vi "Normalize Time Array.vi"(11 "Array Input":dbl[][](array[numeric])) -> (3 "Array Output":dbl[][](array[numeric]))   [LabVIEW 2020]
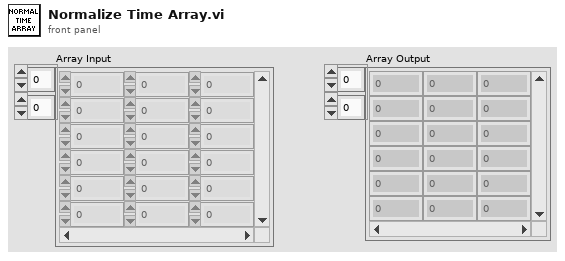
[diagram p1: front panel]
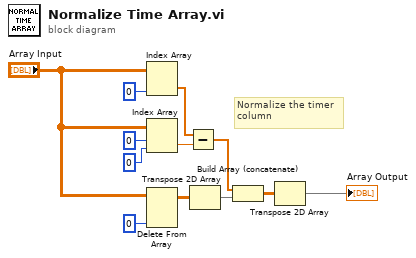
[diagram p0: block diagram]
diagram:
  # "Normalize the timer\ncolumn"
  n1 = Index Array(array="Array Input", index (col)=0 ("disabled index (col)")) -> (element=w7:dbl[])  [unwired: 1 in]
  n2 = Index Array(array="Array Input", index (row)=0 ("disabled index (row)"), index (col)=0 ("disabled index (col)")) -> (element=w6:dbl)
  n3 = Delete From Array(array="Array Input", index (col)=0 ("disabled index (col)")) -> (array with subset deleted=w4:dbl[][])  [unwired: 2 in, 1 out]
  n4 = Subtract(x=w7, y=w6) -> (x-y=w2:dbl[])
  n5 = Transpose 2D Array(2D array=w4) -> (transposed array=w3:dbl[][])
  n6 = Build Array (concatenate)(w2, w3) -> (w1:dbl[][])
  n7 = Transpose 2D Array(2D array=w1) -> (transposed array=→"Array Output":dbl[][])
